vi "constructor.vi"(0 "Parametric in":refnum<class "Parametric.lvclass">, 1 "Color Matrix":dbl[][](array[numeric]), 5 "X Matrix":dbl[][](array[numeric]), 7 "Y Matrix":dbl[][](array[numeric]), 9 "Z Matrix":dbl[][](array[numeric]), 11 "error in (no error)":errorcluster, 12 "Plot ID":i32) -> (4 "Parametric out":refnum<class "Parametric.lvclass">, 15 "error out":errorcluster)   [LabVIEW 2020, in "Parametric.lvclass"]
uses:
  <vilib>/Native 3D Graph/classes/Parametric/Parametric.lvclass
  <vilib>/Native 3D Graph/classes/Parametric/Parametric.lvclass/Parametric.ctl
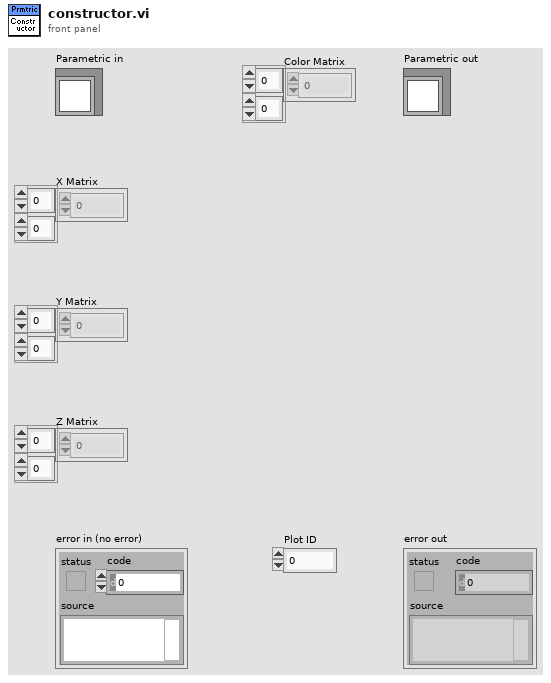
[diagram p1: front panel]
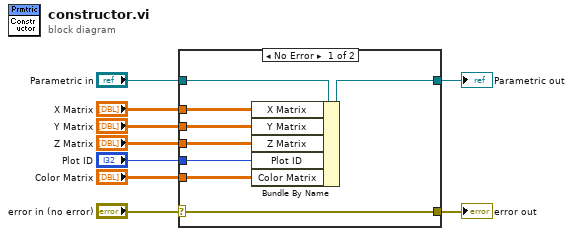
[diagram p0: block diagram]
diagram:
  n1 = case shown="No Error" "error in (no error)" {
    selector: "error in (no error)" -> [w17 w19]
    tunnel: [w17 w19] -> w8
    tunnel: [w15 w18] -> w6
    tunnel: "Parametric in" -> [w16 w18]
    tunnel: "Color Matrix" -> [w14 _]
    tunnel: "X Matrix" -> [w13 _]
    tunnel: "Y Matrix" -> [w12 _]
    tunnel: "Plot ID" -> [w11 _]
    tunnel: "Z Matrix" -> [w10 _]
    frame No Error {
      n2 = Bundle By Name(cluster=w16, "X Matrix"=w13, "Y Matrix"=w12, "Z Matrix"=w10, "Plot ID"=w11, "Color Matrix"=w14) -> (w15:refnum<class "Parametric.lvclass">)
    }
    frame Error {
    }
  }
  "error out" <- w8
  "Parametric out" <- w6
